vi "Frequency Filter.vi"(8 "error in (no error)":errorcluster, 9 "Observed LM Array":T3(array[cluster]), 10 "SLAM In":T1) -> (0 "error out":errorcluster, 2 "SLAM Out":T1)   [LabVIEW 2009]
uses:
  Controls/SLAM.ctl
  <vilib>/Analysis/Matrix/Datatypes/RealMatrix.ctl
  <vilib>/Analysis/Matrix/NI_Matrix.lvlib
panel:
  out "SLAM Out":T1
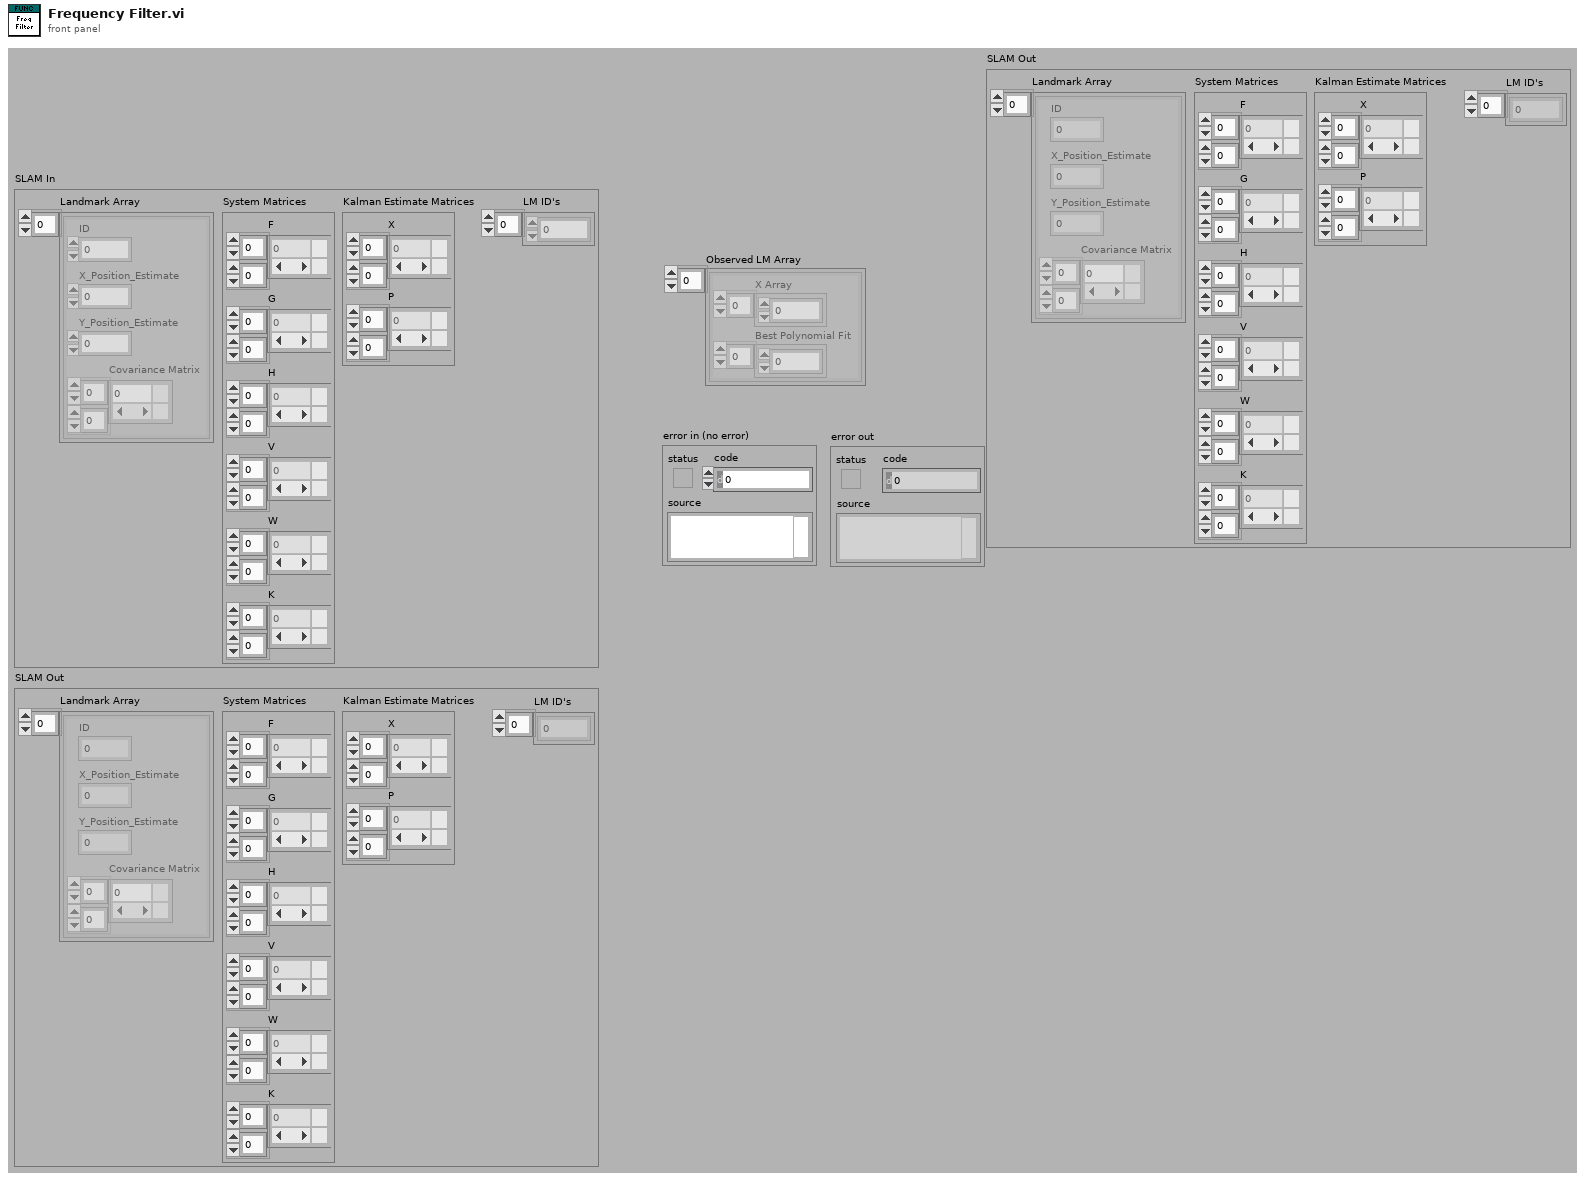
[diagram p1: front panel]
types:
  T1 = typedef "SLAM.ctl" = cluster{"Landmark Array":cluster{"ID":dbl, "X_Position_Estimate":dbl, "Y_Position_Estimate":dbl, "Covariance Matrix":T2}[], "System Matrices":cluster{"F":T2, "G":T2, "H":T2, "V":T2, "W":T2, "K":T2}, "Kalman Estimate Matrices":cluster{"X":T2, "P":T2}, "LM ID's":dbl[]}
  T2 = typedef "NI_Matrix.lvlib/RealMatrix.ctl" = dbl[][]
  T3 = cluster{"X Array":dbl[], "Best Polynomial Fit":dbl[]}[]
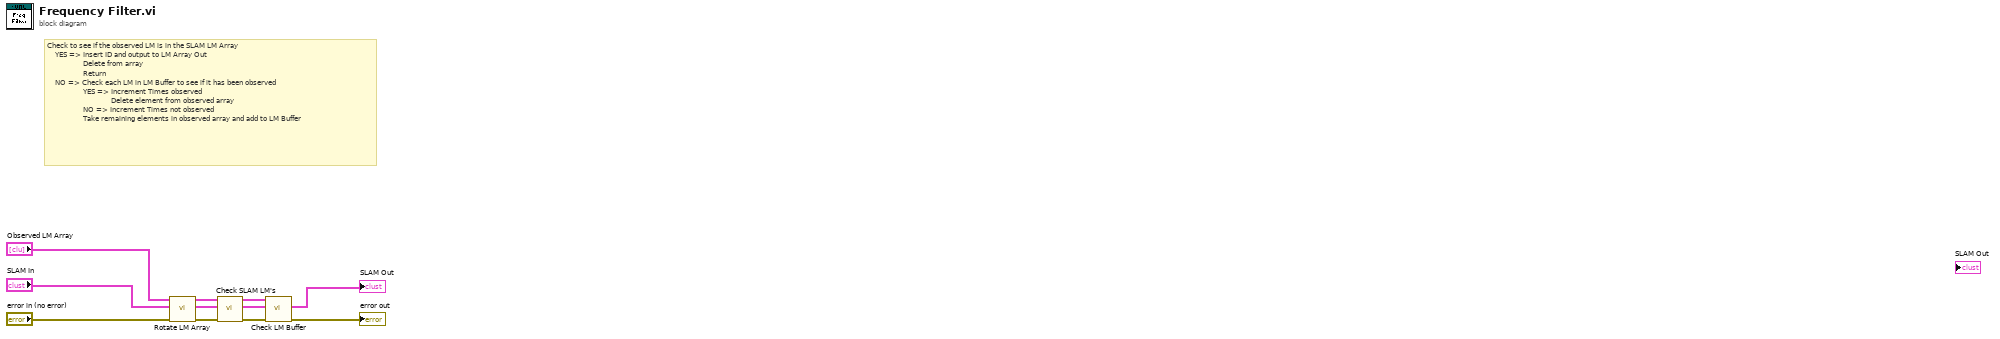
[diagram p0: block diagram]
diagram:
  # "Check to see if the observed LM is in the SLAM LM Array\n    YES => Insert ID and output to LM Array Out\n                  Delete from array\n                  Return\n    NO => Check each LM in LM Buffer to see if it has been observed\n                  YES => Increment Times observed\n                                Delete element from observed array\n                  NO => Increment Times not observed\n                  Take remaining elements in observed array and add to LM Buffer"
  n1 = call "Rotate LM Array.vi"("error in (no error)"="error in (no error)", "SLAM In"="SLAM In", "Observed LM Array"="Observed LM Array") -> ("error out"=w6:errorcluster, "SLAM Out"=w8:T1, "Rotated Observed LM Array"=w7:T3)  [unwired: 6 in]
  n2 = call "Check SLAM LM's.vi"("error in (no error)"=w6, "SLAM In"=w8, "Observed LM Array"=w7) -> ("error out"=w5:errorcluster, "SLAM Out"=w4:T1, "Observed LM Out"=w3:T3)  [unwired: 6 in]
  n3 = call "Check LM Buffer.vi"("error in (no error)"=w5, "SLAM In"=w4, "Observed LM Array"=w3) -> ("error out"=→"error out":errorcluster, "SLAM Out"=→"SLAM Out":T1)  [unwired: 7 in]
